vi "WriteToDigital.vi"(2 "New DO":cluster{"Inst. #":string, "State":bool}[](array[cluster]), 3 "DO in":cluster{"Inst. #":string, "State":bool}[](array[cluster])) -> (1 "DO out":cluster{"Inst. #":string, "State":bool}[](array[cluster]))   [LabVIEW 2020]
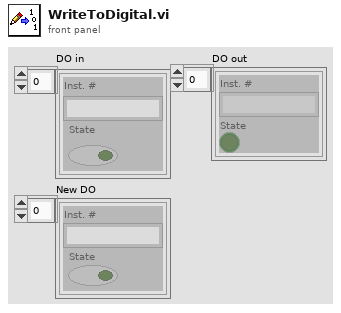
[diagram p1: front panel]
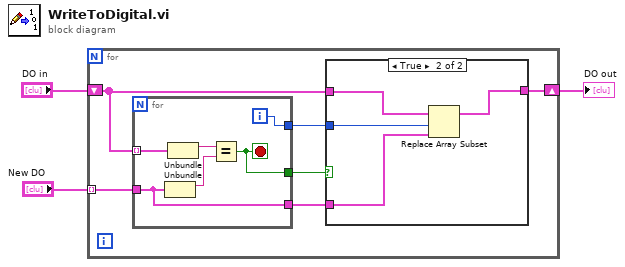
[diagram p0: block diagram]
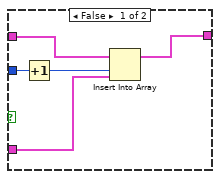
[diagram p2: hidden frame]
diagram:
  n1 = for {
    tunnel: "New DO" -> [w8] mode=indexing
    shift-right: [w6] -> w1
    shift-left: "DO in" -> [w7]
    n2 = for {
      tunnel: [w24] -> w9
      tunnel: w8 -> [w20]
      tunnel: w7 -> [w23] mode=indexing
      tunnel: [w20] -> w5
      tunnel: [w19] -> w4
      i -> [w24]
      stop <- w19 stop-if-true
      n3 = Unbundle(w20) -> ("Inst. #"=w21:string)  [unwired: 1 out]
      n4 = Unbundle(w23) -> ("Inst. #"=w22:string)  [unwired: 1 out]
      n5 = Equal?(x=w22, y=w21) -> (x = y?=w19:bool)
    }
    n6 = case shown="True" w4 {
      tunnel: w9 -> [w14 w18]
      tunnel: w7 -> [w12 w17]
      tunnel: [w10 w16] -> w6
      tunnel: w5 -> [w11 w15]
      frame False {
        n7 = Increment(x=w14) -> (x+1=w13:i32)
        n8 = Insert Into Array(array=w12, index=w13, new element=w11) -> (w10:cluster{"Inst. #":string, "State":bool}[])
      }
      frame True {
        n9 = Replace Array Subset(array=w17, new element=w15, index=w18) -> (w16:cluster{"Inst. #":string, "State":bool}[])
      }
    }
  }
  "DO out" <- w1
